vi "Configure AFG Waveform Period.vi"(8 "error in (no error)":errorcluster, 10 "Period (1E-5 s)":dbl=1e-05, 11 "VISA resource name":refnum<visa-resource-name>) -> (0 "error out":errorcluster, 3 "VISA resource name out":refnum<visa-resource-name>)   [LabVIEW 2016, in "Tektronix DPO MSO 2000 4000 Series.lvlib"]
doc: "Configures the period of the Arbitrary Function Generator waveform, in seconds.\n\n<B>Notes:</B>\n(1) This VI is available for MDO3000 Series only.\n\n(2) Requires the MDO3AFG option to be installed."
uses:
  Tektronix DPO MSO 2000 4000 Series.lvlib
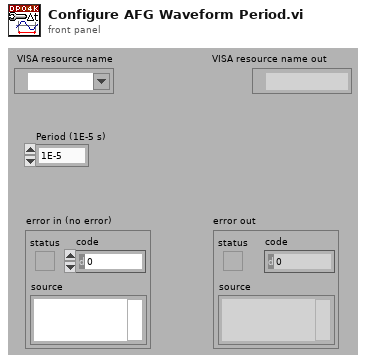
[diagram p1: front panel]
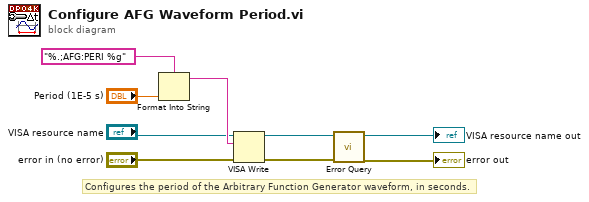
[diagram p0: block diagram]
diagram:
  # "Configures the period of the Arbitrary Function Generator waveform, in seconds."
  n1 = Format Into String(format string="%.;AFG:PERI %g", "Period (1E-5 s)") -> (resulting string=w7:string)  [unwired: 2 in, 1 out]
  n2 = VISA Write(VISA resource name="VISA resource name", write buffer=w7, error in (no error)="error in (no error)") -> (VISA resource name out=w5:refnum<visa-resource-name>, error out=w4:errorcluster)  [unwired: 1 out]
  n3 = call "Error Query.vi"("error in (no error)"=w4, "VISA resource name"=w5) -> ("error out"=→"error out":errorcluster, "VISA resource name out"=→"VISA resource name out":refnum<visa-resource-name>)  [unwired: 6 in, 2 out]
